vi "A170316-11_config.vi"() -> ()   [LabVIEW 2020]
uses:
  Global_Variable/Global.vi
  Database/Global1.vi
  <vilib>/Utility/config.llb/NI_LVConfig.lvlib
panel:
  in  "选项卡控件":enum32{"工艺参数", "追溯码", "备用参数", "产品管理"}(tab)
  in  "操作步骤":T1
  in  "参数设定":string[][](table)
  in  "删除":bool
  in  "确定":bool
  in  "添加":bool
  in  "退出":bool
  in  "更新":bool
  in  "产品型号":string(combo)
  in  "追溯码设定":string[][](table)
  in  "CAN Info":T2={"波特率"=11, "ID"=0, "帧类型"=enum."标准帧", "帧格式"=enum."数据帧", "周期(ms)"=10} caption="CAR_SPEED" {"周期(ms)" min=1 format="%d ms"; "ID" format="0x%x"; "波特率" items=["5Kbps", "10Kbps", "20Kbps", "40Kbps", "50Kbps", "80Kbps", "100Kbps", "125Kbps", "200Kbps", "250Kbps", "400Kbps", "500Kbps", "666Kbps", "800Kbps", "1000Kbps"]}
  in  "CAN_CYCLE":T3(array[cluster]) {"周期(ms)" min=1 format="%d ms"; "ID" format="0x%x"}
  in  "启用CAN":bool
  in  "请输入添加的产品名称":string
  in  "请选择要删除的产品":string(combo)
  # "中间轴装配"
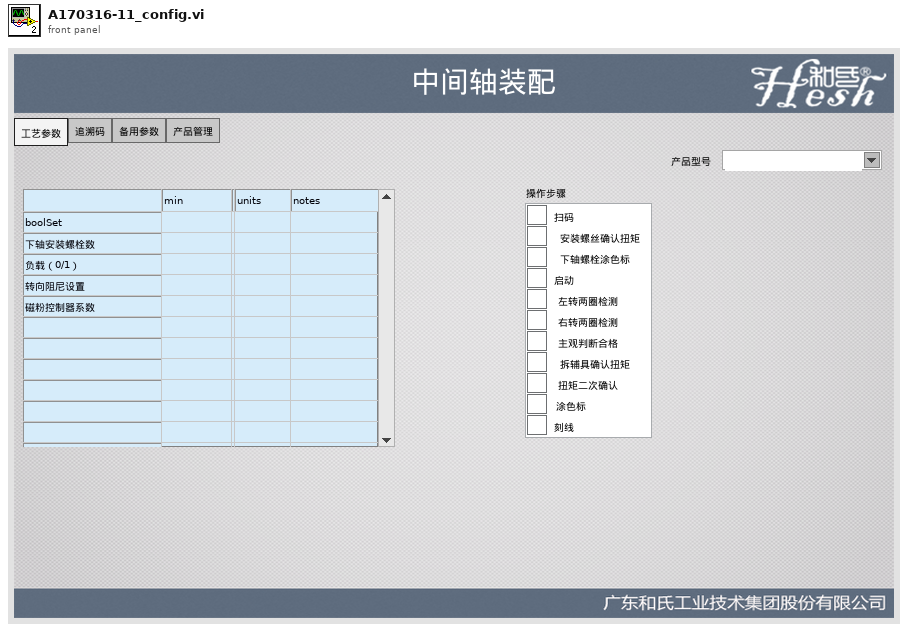
[diagram p1: front panel]
types:
  T1 = cluster{"复选框":bool, "复选框 2":bool, "复选框 11":bool, "复选框 3":bool, "复选框 4":bool, "复选框 5":bool, "复选框 6":bool, "复选框 7":bool, "复选框 8":bool, "复选框 9":bool, "复选框 10":bool}
  T2 = cluster{"波特率":u32, "ID":u32, "帧类型":enum8{"标准帧", "扩展帧"}, "帧格式":enum16{"数据帧", "远程帧"}, "周期(ms)":u32}
  T3 = cluster{"ID":u32, "帧类型":enum8{"标准帧", "扩展帧"}, "帧格式":enum16{"数据帧", "远程帧"}, "帧数据":string, "周期(ms)":u32}[]
  T4 = enum8{"Enabled", "Disabled", "Disabled and Grayed Out"}
  T5 = cluster{"用户编号":string, "用户名":string, "用户密码(密文)":string, "用户权限":string}
  T6 = typedef "NI_LVConfig.lvlib/Config Data RefNum.ctl" = refnum<k1>
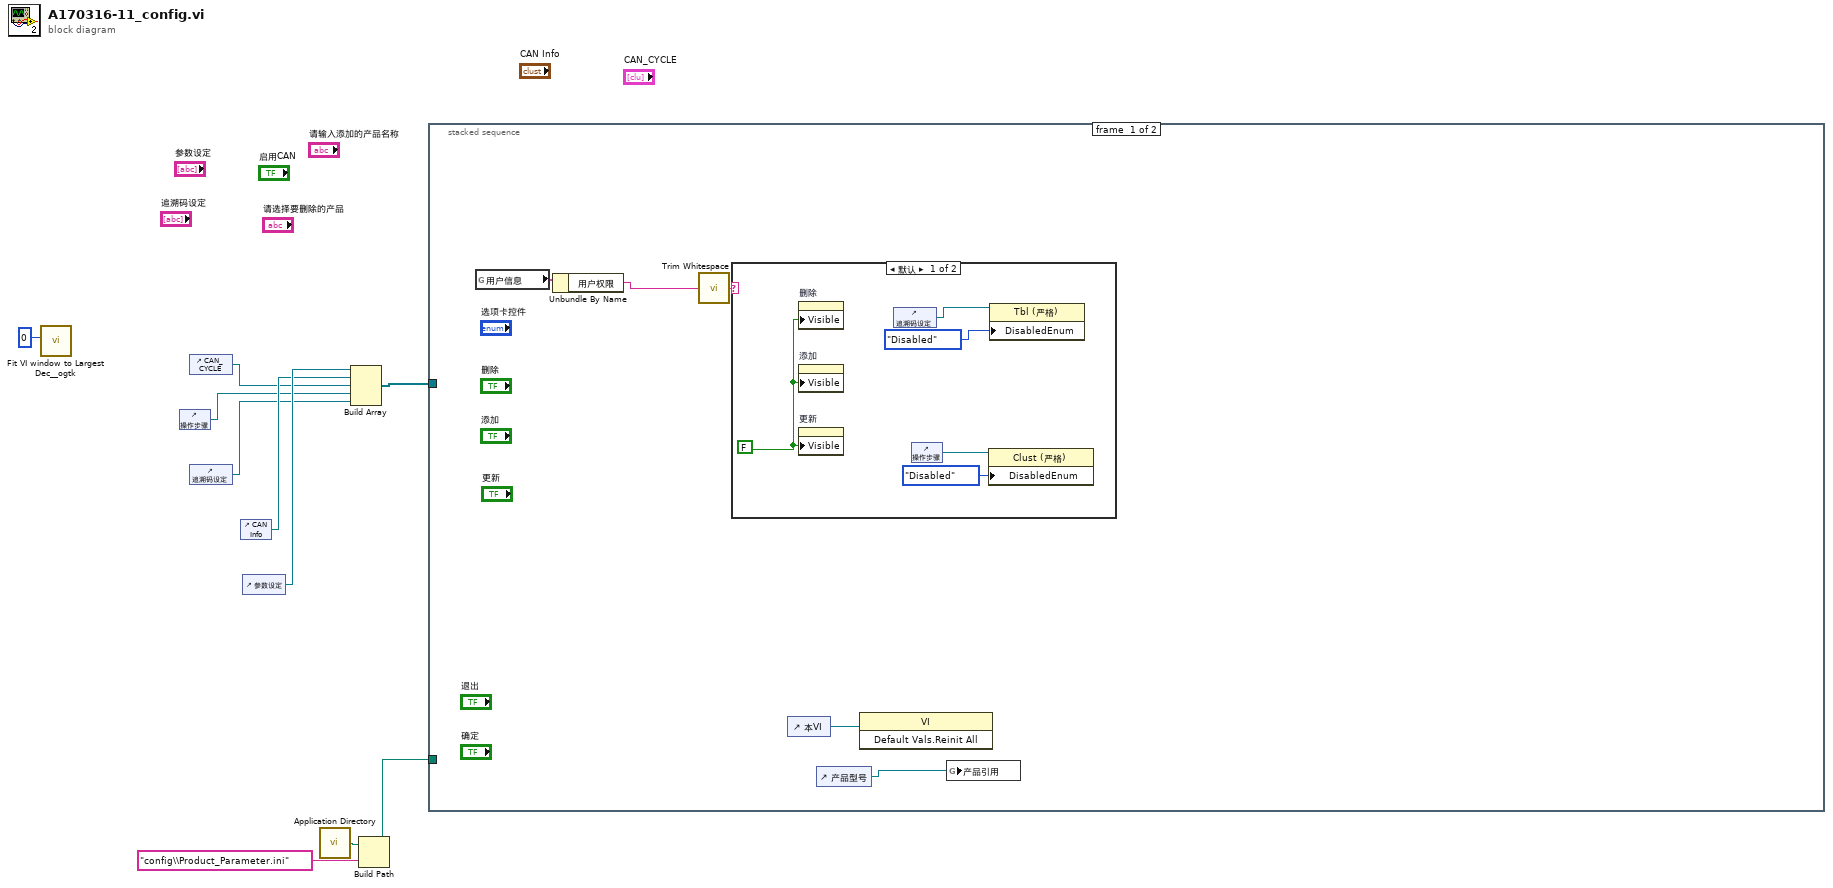
[diagram p0: block diagram]
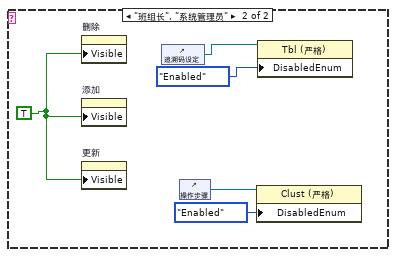
[diagram p2: hidden frame]
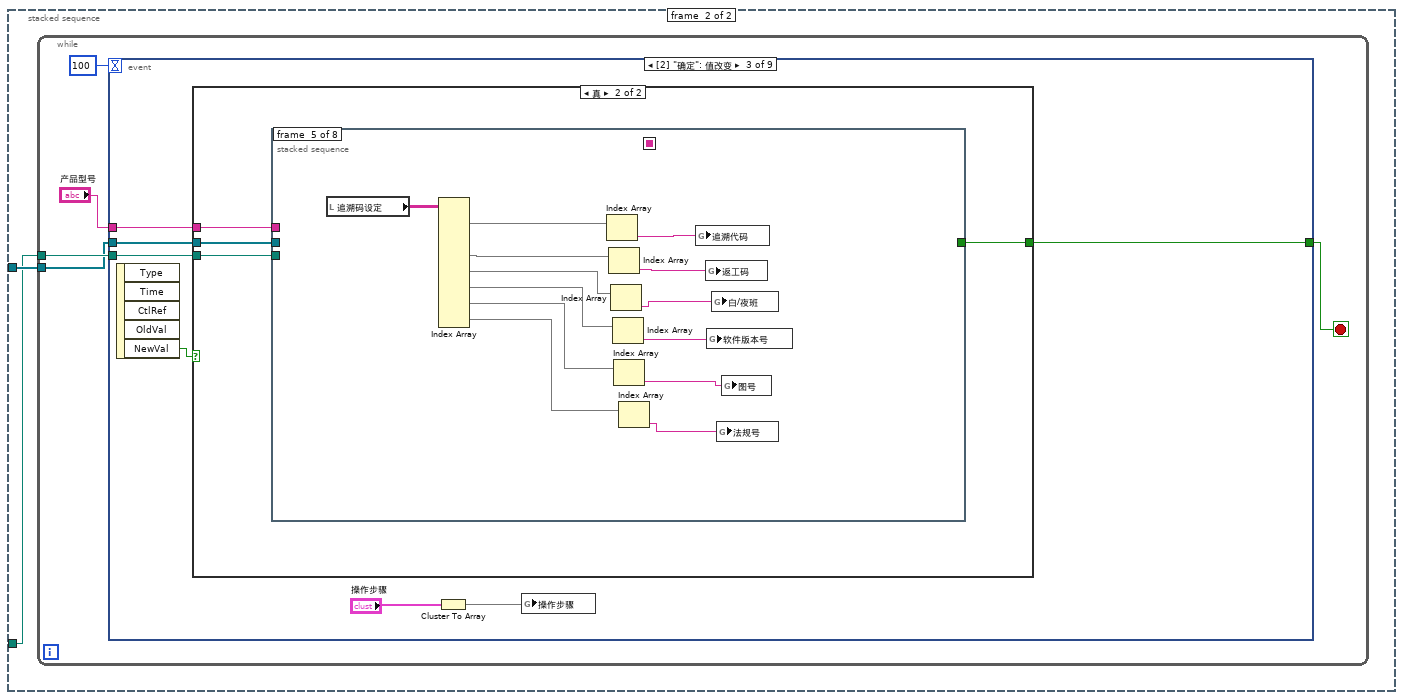
[diagram p3: hidden frame]
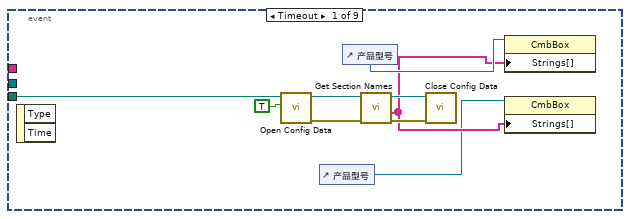
[diagram p4: hidden frame]
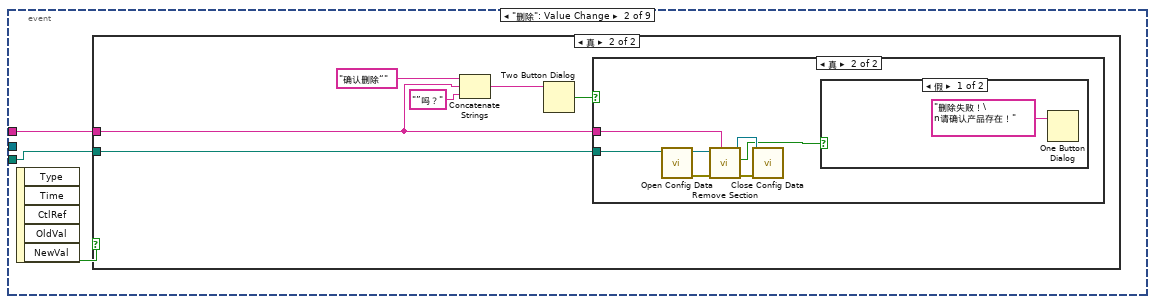
[diagram p5: hidden frame]
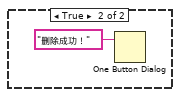
[diagram p8: hidden frame]
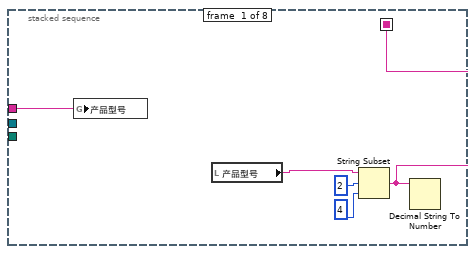
[diagram p10: hidden frame]
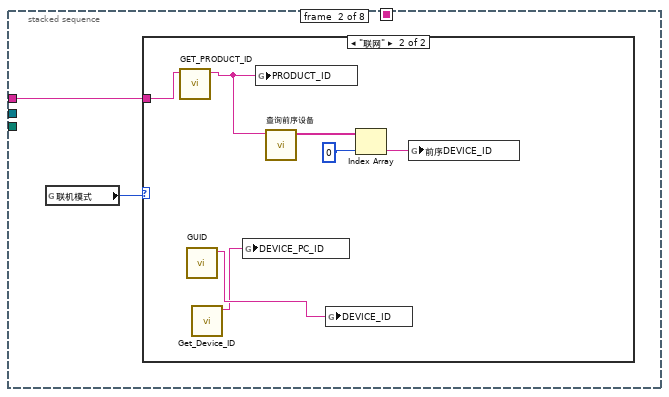
[diagram p11: hidden frame]
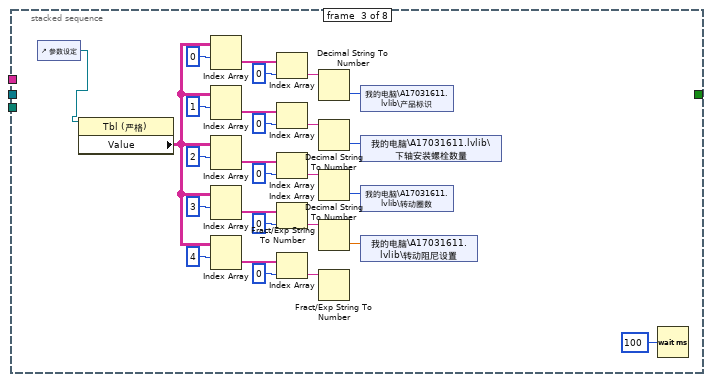
[diagram p13: hidden frame]
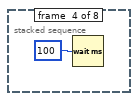
[diagram p14: hidden frame]
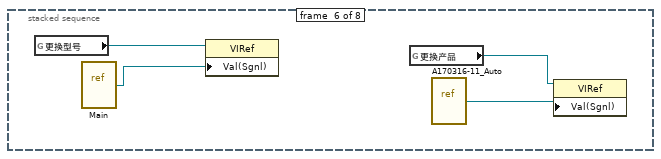
[diagram p15: hidden frame]
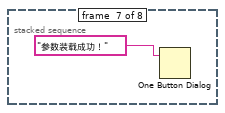
[diagram p16: hidden frame]
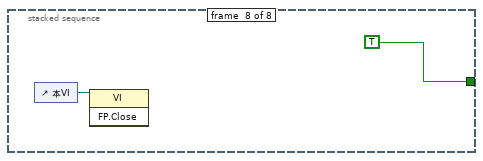
[diagram p17: hidden frame]
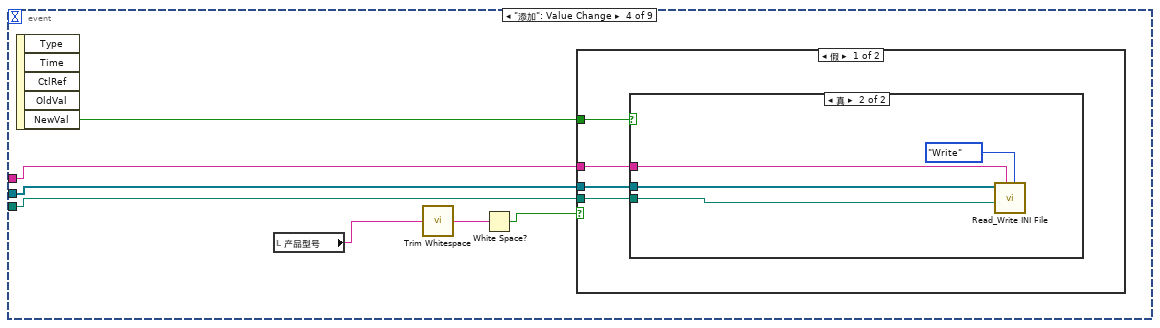
[diagram p18: hidden frame]
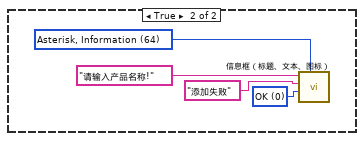
[diagram p20: hidden frame]
diagram:
  n1 = call <userlib>:"Fit VI window to Largest Dec__ogtk.vi"("border spacing (2 px)"=0) -> ()  [unwired: 5 in, 2 out]
  n2 = control-ref of="操作步骤"() -> (w2:refnum<vi>)
  n3 = control-ref of="CAN_CYCLE"() -> (w4:refnum<vi>)
  n4 = control-ref of="追溯码设定"() -> (w1:refnum<vi>)
  n5 = control-ref of="CAN Info"() -> (w5:refnum<vi>)
  n6 = control-ref of="参数设定"() -> (w6:refnum<vi>)
  n7 = call <vilib>:"Application Directory.vi"() -> ("Application Directory"=w10:path)
  n8 = Build Array(w6, w5, w4, w2, w1) -> (w3:refnum<vi>[])
  n9 = Build Path(base path=w10, name or relative path="config\\Product_Parameter.ini" ("名称或相对路径")) -> (appended path=w8:path)
  n10 = stacked-sequence {
    tunnel: w3 -> [_ w27]
    tunnel: w8 -> [_ w26]
    frame #0 {
      n11 = global read "Global1.vi" "用户信息"() -> (w12:T5)
      n12 = Unbundle By Name(w12) -> ("用户权限"=w11:string)
      n13 = call <vilib>:"Trim Whitespace.vi"("string"=w11) -> ("trimmed string"=w15:string)  [unwired: 1 in]
      n14 = case shown="默认" w15 {
        frame Default {
          w20 = FALSE
          n15 = property on="删除" class="Bool (严格)"("Visible"=w20) -> ()  [unwired: 2 in, 2 out]
          n16 = property on="添加" class="Bool (严格)"("Visible"=w20) -> ()  [unwired: 2 in, 2 out]
          n17 = property on="更新" class="Bool (严格)"("Visible"=w20) -> ()  [unwired: 2 in, 2 out]
          n18 = control-ref of="追溯码设定"() -> (w18:refnum<vi>)
          n19 = control-ref of="操作步骤"() -> (w19:refnum<vi>)
          n20 = property class="Clust (严格)"(reference=w19, "DisabledEnum"=T4."Disabled" ("禁用")) -> ()  [unwired: 1 in, 2 out]
          n21 = property class="Tbl (严格)"(reference=w18, "DisabledEnum"=T4."Disabled" ("禁用")) -> ()  [unwired: 1 in, 2 out]
        }
        frame "班组长", "系统管理员" {
          w25 = TRUE
          n22 = property on="删除" class="Bool (严格)"("Visible"=w25) -> ()  [unwired: 2 in, 2 out]
          n23 = property on="添加" class="Bool (严格)"("Visible"=w25) -> ()  [unwired: 2 in, 2 out]
          n24 = property on="更新" class="Bool (严格)"("Visible"=w25) -> ()  [unwired: 2 in, 2 out]
          n25 = control-ref of="追溯码设定"() -> (w22:refnum<vi>)
          n26 = control-ref of="操作步骤"() -> (w24:refnum<vi>)
          n27 = property class="Clust (严格)"(reference=w24, "DisabledEnum"=T4."Enabled" ("禁用")) -> ()  [unwired: 1 in, 2 out]
          n28 = property class="Tbl (严格)"(reference=w22, "DisabledEnum"=T4."Enabled" ("禁用")) -> ()  [unwired: 1 in, 2 out]
        }
      }
      n29 = control-ref of="本VI"() -> (w13:refnum<vi>)
      n30 = control-ref of="产品型号"() -> (w14:refnum<vi>)
      n31 = invoke class="VI" method="Default Vals.Reinit All"(reference=w13) -> ()  [unwired: 2 in, 3 out]
      n32 = global write "Global.vi" "产品引用"(w14) -> ()
    }
    frame #1 {
      n33 = while {
        tunnel: w26 -> [w32]
        tunnel: w27 -> [w30]
        stop <- w31 stop-if-true
        n34 = event shown="[2] \"确定\": 值改变" {
          selector: _ -> [_ _ _ _ _ _ _ _ _]
          dyn-events: _ -> [_ _ _ _ _ _ _ _ _]
          timeout: 100 -> [_ _ _ _ _ _ _ _ _]
          tunnel: w32 -> [w36 w44 w63 w138 w154 _ w171 _ _]
          tunnel: [_ _ w65 _ _ TRUE _ _ TRUE] -> w31
          tunnel: w30 -> [_ _ w64 w139 w155 _ w170 _ _]
          tunnel: "产品型号" -> [_ w42 w62 w133 _ _ _ _ _]
          event Timeout {
            n35 = event-data() -> ()  [unwired: 1 in, 2 out]
            n36 = call <vilib>:"Open Config Data.vi"("create file if necessary (T)"=TRUE, "configuration file path"=w36) -> ("error out"=w38:errorcluster, "refnum"=w37:T6)  [unwired: 7 in, 1 out]
            n37 = control-ref of="产品型号"() -> (w33:refnum<vi>)
            n38 = control-ref of="产品型号"() -> (w35:refnum<vi>)
            n39 = call <vilib>:"Get Section Names.vi"("error in (no error)"=w38, "refnum"=w37) -> ("error out"=w40:errorcluster, "section names"=w34:string[], "refnum out"=w39:T6)  [unwired: 7 in]
            n40 = call <vilib>:"Close Config Data.vi"("error in (no error)"=w40, "refnum"=w39) -> ()  [unwired: 8 in, 2 out]
            n41 = property on="属性节点" class="CmbBox"(reference=w35, "Strings[]"=w34) -> ()  [unwired: 1 in, 2 out]
            n42 = property on="属性节点" class="CmbBox"(reference=w33, "Strings[]"=w34) -> ()  [unwired: 1 in, 2 out]
          }
          event "删除": Value Change {
            n43 = event-data() -> ("NewVal"=w43:bool)  [unwired: 1 in, 4 out]
            n44 = case shown="真" w43 {
              tunnel: w44 -> [_ w46]
              tunnel: w42 -> [_ w45]
              frame False {
              }
              frame True {
                n45 = Concatenate Strings("确认删除“", w45, "”吗？") -> (w48:string)
                n46 = Two Button Dialog(message=w48) -> (T button?=w47:bool)  [unwired: 2 in]
                n47 = case shown="真" w47 {
                  tunnel: w46 -> [_ w52]
                  tunnel: w45 -> [_ w51]
                  frame False {
                  }
                  frame True {
                    n48 = call <vilib>:"Open Config Data.vi"("configuration file path"=w52) -> ("error out"=w54:errorcluster, "refnum"=w57:T6)  [unwired: 8 in, 1 out]
                    n49 = call <vilib>:"Remove Section.vi"("section"=w51, "error in (no error)"=w54, "refnum"=w57) -> ("error out"=w56:errorcluster, "section exists?"=w53:bool, "refnum out"=w55:T6)  [unwired: 6 in]
                    n50 = call <vilib>:"Close Config Data.vi"("error in (no error)"=w56, "refnum"=w55) -> ()  [unwired: 8 in, 2 out]
                    n51 = case shown="假" w53 {
                      frame False {
                        n52 = One Button Dialog(message="删除失败！\n请确认产品存在！" ("消息")) -> ()  [unwired: 1 in, 1 out]
                      }
                      frame True {
                        n53 = One Button Dialog(message="删除成功！" ("消息")) -> ()  [unwired: 1 in, 1 out]
                      }
                    }
                  }
                }
              }
            }
          }
          event "确定": Value Change {
            n54 = event-data() -> ("NewVal"=w66:bool)  [unwired: 1 in, 4 out]
            n55 = case shown="真" w66 {
              tunnel: [_ w70] -> w65
              tunnel: w64 -> [_ w69]
              tunnel: w63 -> [_ w68]
              tunnel: w62 -> [_ w67]
              frame False {
              }
              frame True {
                n56 = stacked-sequence {
                  seq-local: [w75 _ _ _ _ _ _ _] -> [_ _ _ _ _ _ _ _]
                  tunnel: [_ _ _ _ _ _ _ TRUE] -> w70
                  tunnel: w69 -> [_ _ _ _ _ _ _ _]
                  tunnel: w68 -> [_ _ _ _ _ _ _ _]
                  tunnel: w67 -> [w71 w77 _ _ _ _ _ _]
                  frame #0 {
                    n57 = global write "Global.vi" "产品型号"(w71) -> ()
                    n58 = local read "产品型号"() -> (w74:string)
                    n59 = String Subset(string=w74, offset (0)=u16 2 ("偏移量(0)"), length (rest)=u16 4 ("长度（剩余）")) -> (substring=w75:string)
                    n60 = Decimal String To Number(string=w75) -> ()  [unwired: 2 in, 2 out]
                  }
                  frame #1 {
                    n61 = global read "Global1.vi" "联机模式"() -> (w76:enum16{"单机", "联网"})
                    n62 = case shown="\"联网\"" w76 {
                      tunnel: w77 -> [_ w80]
                      frame "单机", Default {
                      }
                      frame "联网" {
                        n63 = call "GET_PRODUCT_ID.vi"("PRODFUCT_NAME"=w80) -> ("PRODUCT_ID"=w84:string)  [unwired: 10 in]
                        n64 = call "GUID.vi"() -> ("trimmed string"=w79:string)  [unwired: 11 in]
                        n65 = call "Get_Device_ID.vi"() -> ("Device_ID"=w78:string)  [unwired: 10 in, 1 out]
                        n66 = global write "Global1.vi" "DEVICE_PC_ID"(w78) -> ()
                        n67 = global write "Global1.vi" "PRODUCT_ID"(w84) -> ()
                        n68 = call "查询前序设备.vi"("PRODUCT_ID"=w84) -> ("前序工位"=w83:string[])  [unwired: 10 in]
                        n69 = global write "Global1.vi" "DEVICE_ID"(w79) -> ()
                        n70 = Index Array(array=w83, index=0 ("索引")) -> (element=w81:string)
                        n71 = global write "Global1.vi" "前序DEVICE_ID"(w81) -> ()
                      }
                    }
                  }
                  frame #2 {
                    n72 = control-ref of="参数设定"() -> (w85:refnum<vi>)
                    n73 = property class="Tbl (严格)"(reference=w85) -> ("Value"=w101:string[][])  [unwired: 1 in, 2 out]
                    n74 = Index Array(array=w101, index (row)=0 ("索引 (行)")) -> (element=w109:string[])  [unwired: 1 in]
                    n75 = Index Array(array=w101, index (row)=1 ("索引 (行)")) -> (element=w94:string[])  [unwired: 1 in]
                    n76 = Index Array(array=w101, index (row)=2 ("索引 (行)")) -> (element=w93:string[])  [unwired: 1 in]
                    n77 = Index Array(array=w101, index (row)=3 ("索引 (行)")) -> (element=w86:string[])  [unwired: 1 in]
                    n78 = Index Array(array=w101, index (row)=4 ("索引 (行)")) -> (element=w87:string[])  [unwired: 1 in]
                    n79 = Index Array(array=w109, index=0 ("索引")) -> (element=w110:string)
                    n80 = Index Array(array=w94, index=0 ("索引")) -> (element=w98:string)
                    n81 = Index Array(array=w93, index=0 ("索引")) -> (element=w97:string)
                    n82 = Index Array(array=w86, index=0 ("索引")) -> (element=w90:string)
                    n83 = Index Array(array=w87, index=0 ("索引")) -> (element=w88:string)
                    n84 = Decimal String To Number(string=w110) -> (number=w107:i32)  [unwired: 2 in, 1 out]
                    n85 = Decimal String To Number(string=w98) -> (number=w100:i32)  [unwired: 2 in, 1 out]
                    n86 = Decimal String To Number(string=w97) -> (number=w95:i32)  [unwired: 2 in, 1 out]
                    n87 = Fract/Exp String To Number(string=w90) -> (number=w89:dbl)  [unwired: 3 in, 1 out]
                    n88 = Fract/Exp String To Number(string=w88) -> ()  [unwired: 3 in, 2 out]
                    n89 = shared-variable "我的电脑\\A17031611.lvlib\\产品标识"(w107) -> ()  [unwired: 1 in, 1 out]
                    n90 = shared-variable "我的电脑\\A17031611.lvlib\\下轴安装螺栓数量"(w100) -> ()  [unwired: 1 in, 1 out]
                    n91 = shared-variable "我的电脑\\A17031611.lvlib\\转动圈数"(w95) -> ()  [unwired: 1 in, 1 out]
                    n92 = shared-variable "我的电脑\\A17031611.lvlib\\转动阻尼设置"(w89) -> ()  [unwired: 1 in, 1 out]
                    n93 = Wait (ms)(milliseconds to wait=u32 100) -> ()  [unwired: 1 out]
                  }
                  frame #3 {
                    n94 = Wait (ms)(milliseconds to wait=u32 100) -> ()  [unwired: 1 out]
                  }
                  frame #4 {
                    n95 = local read "追溯码设定"() -> (w125:string[][])
                    n96 = Index Array(array=w125) -> (element #1=w124:string[], element #3=w122:string[], element #4=w120:string[], element #5=w118:string[], element #6=w116:string[], element #7=w115:string[])  [unwired: 14 in, 1 out]
                    n97 = Index Array(array=w124) -> (element=w123:string)  [unwired: 1 in]
                    n98 = Index Array(array=w122) -> (element=w121:string)  [unwired: 1 in]
                    n99 = Index Array(array=w120) -> (element=w119:string)  [unwired: 1 in]
                    n100 = Index Array(array=w118) -> (element=w117:string)  [unwired: 1 in]
                    n101 = Index Array(array=w116) -> (element=w114:string)  [unwired: 1 in]
                    n102 = Index Array(array=w115) -> (element=w113:string)  [unwired: 1 in]
                    n103 = global write "Global.vi" "追溯代码"(w123) -> ()
                    n104 = global write "Global.vi" "返工码"(w121) -> ()
                    n105 = global write "Global.vi" "软件版本号"(w117) -> ()
                    n106 = global write "Global.vi" "白/夜班"(w119) -> ()
                    n107 = global write "Global.vi" "法规号"(w113) -> ()
                    n108 = global write "Global.vi" "图号"(w114) -> ()
                  }
                  frame #5 {
                    n109 = global read "Global.vi" "更换型号"() -> (w127:refnum<vi>)
                    n110 = vi-ref "Main.vi"() -> (w126:refnum<vi>)
                    n111 = property class="VIRef"(reference=w127, "Val(Sgnl)"=w126) -> ()  [unwired: 1 in, 2 out]
                    n112 = global read "Global.vi" "更换产品"() -> (w129:refnum<vi>)
                    n113 = vi-ref "A170316-11_Auto.vi"() -> (w128:refnum<vi>)
                    n114 = property class="VIRef"(reference=w129, "Val(Sgnl)"=w128) -> ()  [unwired: 1 in, 2 out]
                  }
                  frame #6 {
                    n115 = One Button Dialog(message="参数装载成功！" ("消息")) -> ()  [unwired: 1 in, 1 out]
                  }
                  frame #7 {
                    n116 = control-ref of="本VI"() -> (w131:refnum<vi>)
                    n117 = invoke class="VI" method="FP.Close"(reference=w131) -> ()  [unwired: 2 in, 3 out]
                  }
                }
              }
            }
            n118 = Cluster To Array(cluster="操作步骤") -> (array=w60:bool[])
            n119 = global write "Global.vi" "操作步骤"(w60) -> ()
          }
          event "添加": Value Change {
            n120 = event-data() -> ("NewVal"=w137:bool)  [unwired: 1 in, 4 out]
            n121 = local read "产品型号"() -> (w134:string)
            n122 = call <vilib>:"Trim Whitespace.vi"("string"=w134) -> ("trimmed string"=w135:string)  [unwired: 1 in]
            n123 = White Space?(1:w135) -> (0:w136:bool)
            n124 = case shown="假" w136 {
              tunnel: w139 -> [w143 _]
              tunnel: w138 -> [w142 _]
              tunnel: w137 -> [w141 _]
              tunnel: w133 -> [w140 _]
              frame False {
                n125 = case shown="真" w141 {
                  tunnel: w143 -> [_ w144]
                  tunnel: w142 -> [_ w147]
                  tunnel: w140 -> [_ w145]
                  frame False {
                  }
                  frame True {
                    n126 = call "Read_Write INI File.vi"("Mode"=enum16{"Read", "Write"}."Write", "Section"=w145, "Filepath"=w147, "Ctl Refnum"=w144) -> ()  [unwired: 7 in, 1 out]
                  }
                }
              }
              frame True {
                w148 = 64 items=["None"=0, "Hand, Error, Stop"=16, "Question"=32, "Exclamation, Warning"=48, "Asterisk, Information"=64] ("icon")
                w149 = 0 items=["OK", "OKCancel", "AbortRetryIgnore", "YesNoCancel", "YesNo", "RetryCancel"] ("buttons")
                n127 = call "信息框（标题、文本、图标）.vi"("icon"=w148, "buttons"=w149, "caption"="添加失败", "text"="请输入产品名称!") -> ()  [unwired: 6 in, 2 out]
              }
            }
          }
          event "产品型号": Value Change {
            n128 = event-data() -> ("CtlRef"=w153:refnum<vi>, "NewVal"=w152:string)  [unwired: 1 in, 3 out]
            n129 = stacked-sequence {
              tunnel: w155 -> [_ w161]
              tunnel: w154 -> [_ w164]
              tunnel: w153 -> [w157 _]
              tunnel: w152 -> [w156 _]
              frame #0 {
                n130 = stacked-sequence {
                  tunnel: w157 -> [_ w159]
                  tunnel: w156 -> [_ w160]
                  frame #0 {
                    n131 = control-ref of="This VI"() -> (w158:refnum<vi>)
                    n132 = invoke class="VI" method="Default Vals.Reinit All"(reference=w158) -> ()  [unwired: 2 in, 3 out]
                  }
                  frame #1 {
                    n133 = property class="CmbBox"(reference=w159, "Value"=w160) -> ()  [unwired: 1 in, 2 out]
                  }
                }
              }
              frame #1 {
                n134 = local read "产品型号"() -> (w162:string)
                n135 = call "Read_Write INI File.vi"("Mode"=enum16{"Read", "Write"}."Read", "Section"=w162, "Filepath"=w164, "Ctl Refnum"=w161) -> ()  [unwired: 7 in, 1 out]
              }
            }
          }
          event "退出": Value Change {
            n136 = event-data() -> ()  [unwired: 1 in, 5 out]
            n137 = control-ref of="本VI"() -> (w167:refnum<vi>)
            n138 = invoke class="VI" method="FP.Close"(reference=w167) -> (reference out=w165:refnum<vi>, error out=w166:errorcluster)  [unwired: 2 in, 1 out]
            n139 = Close Reference(reference=w165, error in (no error)=w166) -> ()  [unwired: 1 out]
          }
          event "更新": Value Change {
            n140 = event-data() -> ("NewVal"=w169:bool)  [unwired: 1 in, 4 out]
            n141 = case shown="真" w169 {
              tunnel: w171 -> [_ w176]
              tunnel: w170 -> [_ w172]
              frame False {
              }
              frame True {
                n142 = local read "产品型号"() -> (w174:string)
                n143 = call "Read_Write INI File.vi"("Mode"=enum16{"Read", "Write"}."Write", "Section"=w174, "Filepath"=w176, "Ctl Refnum"=w172) -> ("error out"=w175:errorcluster)  [unwired: 7 in]
                n144 = case shown="无错误" w175 {
                  frame No Error {
                    n145 = call "浮动通知.vi"("通知内容"="更新成功！") -> ()  [unwired: 11 in]
                  }
                  frame Error {
                    n146 = call "浮动通知.vi"("通知内容"="更新失败！") -> ()  [unwired: 11 in]
                  }
                }
              }
            }
          }
          event "请输入添加的产品名称": Value Change {
            n147 = event-data() -> ("OldVal"=w181:string)  [unwired: 1 in, 5 out]
            n148 = control-ref of="产品型号"() -> (w179:refnum<vi>)
            n149 = property on="属性节点" class="CmbBox"(reference=w179) -> ("Strings[]"=w180:string[])  [unwired: 1 in, 2 out]
            n150 = for {
              tunnel: w181 -> [w182]
              tunnel: w180 -> [w183] mode=indexing
              n151 = Equal?(x=w182, y=w183) -> (x = y?=w184:bool)
              n152 = case shown="真" w184 {
                tunnel: w182 -> [_ w185]
                frame False {
                }
                frame True {
                  n153 = stacked-sequence {
                    tunnel: w185 -> [w191 _]
                    frame #0 {
                      w186 = 64 items=["None"=0, "Hand, Error, Stop"=16, "Question"=32, "Exclamation, Warning"=48, "Asterisk, Information"=64] ("icon")
                      w187 = 0 items=["OK", "OKCancel", "AbortRetryIgnore", "YesNoCancel", "YesNo", "RetryCancel"] ("buttons")
                      n154 = Concatenate Strings("已经存在产品”" ("text"), w191, "“\n请勿重复添加！" ("字符串")) -> (w189:string)
                      n155 = call "信息框（标题、文本、图标）.vi"("icon"=w186, "buttons"=w187, "caption"="产品重复", "text"=w189) -> ()  [unwired: 6 in, 2 out]
                    }
                    frame #1 {
                      n156 = local write "请输入添加的产品名称"("" ("请输入添加的产品名称")) -> ()
                    }
                  }
                }
              }
            }
          }
          event Panel Close {
            n157 = event-data() -> ()  [unwired: 1 in, 3 out]
          }
        }
      }
    }
  }
